vi "Save-configuration-with-dialog.vi"(8 "error in (no error)":errorcluster, 11 "Object ref in":T1) -> (0 "error out":errorcluster, 1 "Succes?":bool, 3 "Object ref out":T1)   [LabVIEW 2013, in "HardwareCharacterization.lvlib" / "HC-Main.lvclass"]
uses:
  HC-Main.lvclass
  Object-reference.ctl
  HC-Main.lvclass/HC-Main.ctl
  Configuration-data.ctl
  Options.ctl
  Read Status.vi
  Read Option 1.vi
  <vilib>/Utility/xml.llb/Write to XML File(string).vi
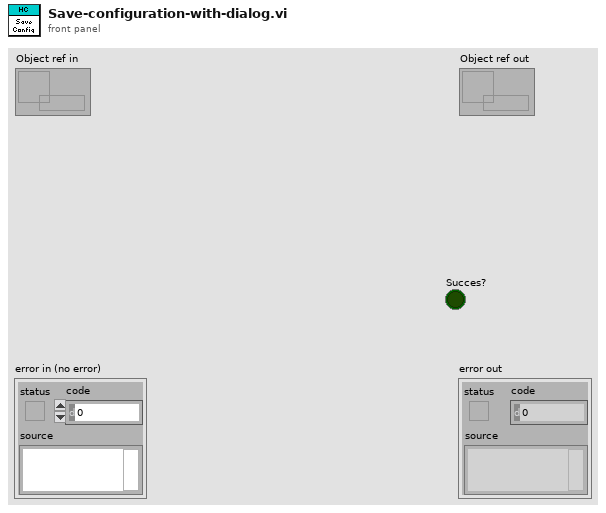
[diagram p1: front panel]
types:
  T1 = typedef "HardwareCharacterization.lvlib/HC-Main.lvclass/Object-reference.ctl" = refnum<data-value>
  T2 = typedef "HardwareCharacterization.lvlib/HC-Main.lvclass/Configuration-data.ctl" = cluster{"Options":T3}
  T3 = typedef "HardwareCharacterization.lvlib/HC-Main.lvclass/Options.ctl" = cluster{"Option 1":bool}
  T4 = typedef "HardwareCharacterization.lvlib/HC-Main.lvclass/Application-status.ctl" = enum16{"Idle", "Initialized", "Configured", "Activated", "Started", "Paused", "Stopped", "Reset", "Error", "Exited"}
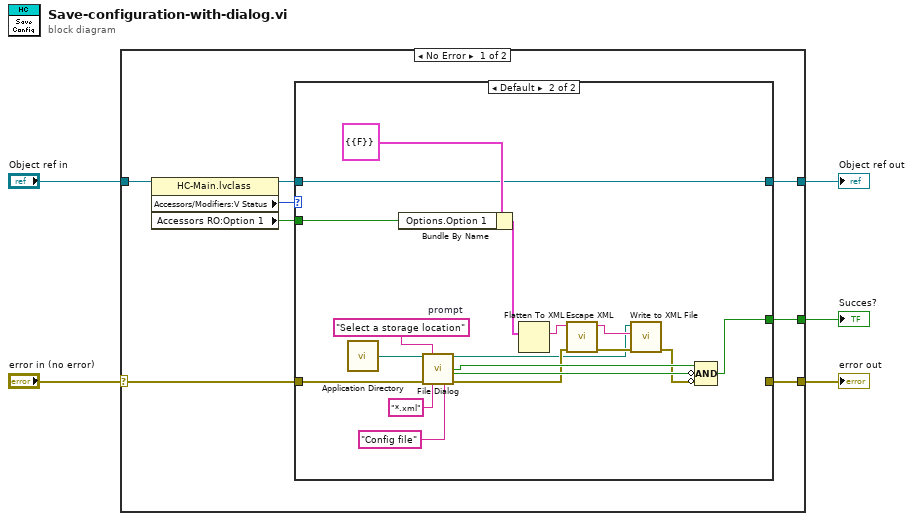
[diagram p0: block diagram]
diagram:
  n1 = case shown="No Error" "error in (no error)" {
    selector: "error in (no error)" -> [w13 w35]
    tunnel: [w10 w35] -> w4
    tunnel: [w9 w34] -> w2
    tunnel: "Object ref in" -> [w12 w34]
    tunnel: [w6 _] -> w1
    frame No Error {
      n2 = property class="HC-Main.lvclass"(reference=w12) -> (reference out=w11:T1, "Accessors/Modifiers:V Status"=w8:T4, "Accessors RO:Option 1"=w7:bool)  [unwired: 1 in, 1 out]
      n3 = case shown="Default" w8 {
        tunnel: w13 -> [w15 w30]
        tunnel: w11 -> [w14 w17]
        tunnel: [w15 _] -> w10
        tunnel: [w14 w17] -> w9
        tunnel: w7 -> [_ w26]
        tunnel: [_ w16] -> w6
        frame "Error" {
        }
        frame Default {
          w32 = "Select a storage location"  # prompt
          n4 = call <vilib>:"Application Directory.vi"() -> ("Application Directory"=w33:path)
          n5 = Bundle By Name(cluster=T2 {"Options"={"Option 1"=FALSE}} ("Configuration data"), "Options.Option 1"=w26) -> (w21:T2)
          n6 = call "File Dialog"("start path"=w33, "prompt"=w32, "error in"=w30, "pattern (all files)"="*.xml", "pattern label"="Config file") -> ("selected path"=w18:path, "exists"=w28:bool, "cancelled"=w27:bool, "error out"=w20:errorcluster)  [unwired: 7 in]
          n7 = Flatten To XML(anything=w21) -> (xml string=w24:string)
          n8 = call <vilib>:"Escape XML.vi"("error in (no error)"=w20, "XML String In"=w24) -> ("error out"=w23:errorcluster, "XML String Out"=w22:string)  [unwired: 8 in]
          n9 = call-poly <vilib>:"Write to XML File.vi"("error in (no error)"=w23, "XML Input"=w22, "XML File Path"=w18) -> ("error out"=w19:errorcluster)  [unwired: 6 in, 2 out]
          n10 = Compound Arithmetic op=AND(w28, invert w27, invert w19) -> (w16:bool)
        }
      }
    }
    frame Error {
    }
  }
  "error out" <- w4
  "Object ref out" <- w2
  "Succes?" <- w1
